vi "start_vlc_1.vi"(6 "Filename":string, 7 "wait until completion? (F)":bool, 8 "error in (no error)":errorcluster, 9 "Operation":T1(ring)=enum."Preview 320x240", 10 "VLC command":string="dshow:// --run-time=20 :dshow-vdev=\"\" :dshow-adev=\"none\" :dshow-caching=80 :dshow-fps=30.000000 -I http :sout=#transcode{vcodec=mp1v,vb=2048}:duplicate{dst=std{access=file,mux=mpeg1,dst=\"FILENAME.mpg\"}} vlc://quit", 11 "video_capture_dir":path) -> (0 "error out":errorcluster, 1 "standard output":string, 3 "standard error":string)   [LabVIEW 2018]
panel:
  out "VLC command Submitted":string
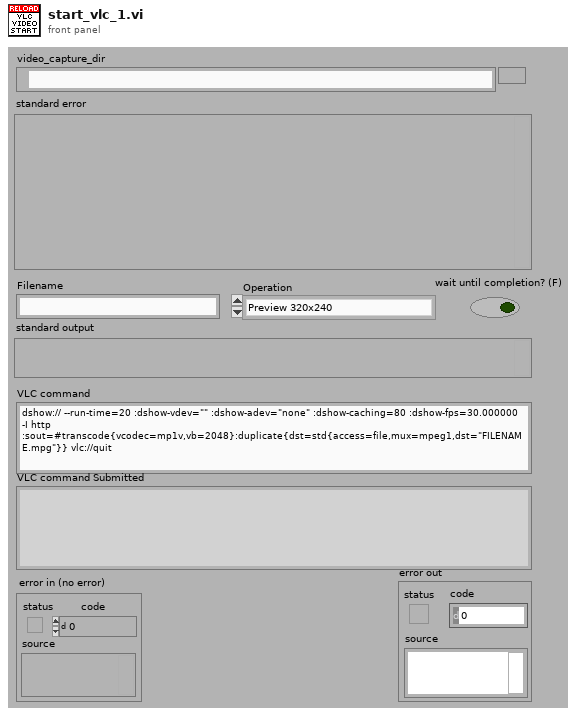
[diagram p1: front panel]
types:
  T1 = enum16{"Record to File", "Preview 320x240", "Preview 640x480"}
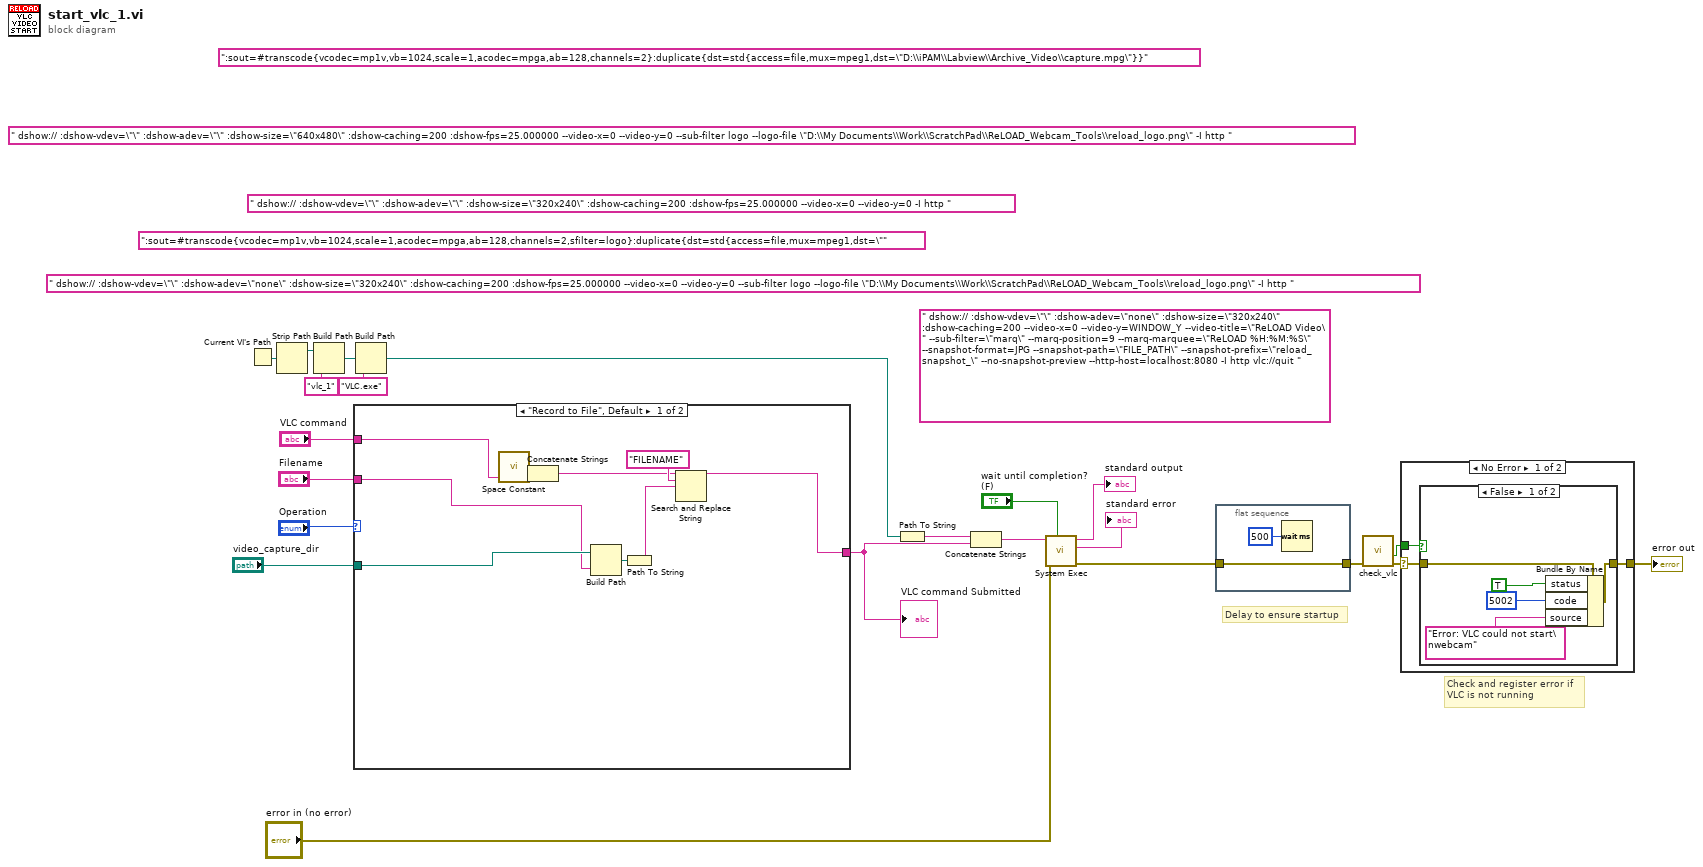
[diagram p0: block diagram]
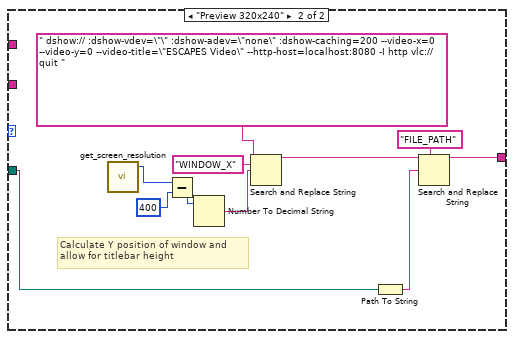
[diagram p4: hidden frame]
diagram:
  (unwired) " dshow:// :dshow-vdev=\"\" :dshow-adev=\"none\" :dshow-size=\"320x240\" :dshow-caching=200 --video-x=0 --video-y=WINDOW_Y --video-title=\"ReLOAD Video\" --sub-filter=\"marq\" --marq-position=9 --marq-marquee=\"ReLOAD %H:%M:%S\" --snapshot-format=JPG --snapshot-path=\"FILE_PATH\" --snapshot-prefix=\"reload_snapshot_\" --no-snapshot-preview --http-host=localhost:8080 -I http vlc://quit " ("Image Name")
  (unwired) ":sout=#transcode{vcodec=mp1v,vb=1024,scale=1,acodec=mpga,ab=128,channels=2}:duplicate{dst=std{access=file,mux=mpeg1,dst=\"D:\\iPAM\\Labview\\Archive_Video\\capture.mpg\"}}" ("Image Name")
  (unwired) ":sout=#transcode{vcodec=mp1v,vb=1024,scale=1,acodec=mpga,ab=128,channels=2,sfilter=logo}:duplicate{dst=std{access=file,mux=mpeg1,dst=\"" ("Image Name")
  (unwired) " dshow:// :dshow-vdev=\"\" :dshow-adev=\"none\" :dshow-size=\"320x240\" :dshow-caching=200 :dshow-fps=25.000000 --video-x=0 --video-y=0 --sub-filter logo --logo-file \"D:\\My Documents\\Work\\ScratchPad\\ReLOAD_Webcam_Tools\\reload_logo.png\" -I http " ("Image Name")
  (unwired) " dshow:// :dshow-vdev=\"\" :dshow-adev=\"\" :dshow-size=\"640x480\" :dshow-caching=200 :dshow-fps=25.000000 --video-x=0 --video-y=0 --sub-filter logo --logo-file \"D:\\My Documents\\Work\\ScratchPad\\ReLOAD_Webcam_Tools\\reload_logo.png\" -I http " ("Image Name")
  (unwired) " dshow:// :dshow-vdev=\"\" :dshow-adev=\"\" :dshow-size=\"320x240\" :dshow-caching=200 :dshow-fps=25.000000 --video-x=0 --video-y=0 -I http " ("Image Name")
  # "Check and register error if\nVLC is not running"
  # "Delay to ensure startup"
  n1 = Current VI's Path() -> (path=w16:path)
  n2 = Strip Path(path=w16) -> (stripped path=w15:path)  [unwired: 1 out]
  n3 = Build Path(base path=w15, name or relative path="vlc_1" ("search string")) -> (appended path=w13:path)
  n4 = case shown="\"Record to File\", Default" "Operation" {
    tunnel: [w23 w35] -> w10
    tunnel: "video_capture_dir" -> [w26 w36]
    tunnel: "Filename" -> [w25 _]
    tunnel: "VLC command" -> [w24 _]
    frame "Record to File", Default {
      n5 = call <vilib>:"Space Constant.vi"() -> ("String"=w27:string)
      n6 = Concatenate Strings(w27, w24) -> (w28:string)
      n7 = Build Path(base path=w26, name or relative path=w25) -> (appended path=w29:path)
      n8 = Path To String(path=w29) -> (string=w30:string)
      n9 = Search and Replace String(input string=w28, search string="FILENAME", replace string=w30) -> (result string=w23:string)  [unwired: 1 in, 7 out]
    }
    frame "Preview 320x240" {
      # "Calculate Y position of window and\nallow for titlebar height"
      n10 = call "get_screen_resolution.vi"() -> ("Width pixels"=w33:i16)  [unwired: 5 out]
      n11 = Subtract(x=w33, y=400) -> (x-y=w40:i32)
      n12 = Number To Decimal String(number=w40) -> (decimal integer string=w41:string)  [unwired: 1 out]
      n13 = Search and Replace String(input string=" dshow:// :dshow-vdev=\"\" :dshow-adev=\"none\" :dshow-caching=200 --video-x=0 --video-y=0 --video-title=\"ESCAPES Video\" --http-host=localhost:8080 -I http vlc://quit " ("Image Name"), search string="WINDOW_X", replace string=w41) -> (result string=w32:string)  [unwired: 1 in, 7 out]
      n14 = Path To String(path=w36) -> (string=w37:string)
      n15 = Search and Replace String(input string=w32, search string="FILE_PATH", replace string=w37) -> (result string=w35:string)  [unwired: 1 in, 7 out]
    }
  }
  "VLC command Submitted" <- w10
  n16 = Build Path(base path=w13, name or relative path="VLC.exe" ("search string")) -> (appended path=w12:path)
  n17 = Path To String(path=w12) -> (string=w20:string)
  n18 = Concatenate Strings(w20, w10) -> (w21:string)
  n19 = call <vilib>:"System Exec.vi"("wait until completion? (T)"="wait until completion? (F)", "error in (no error)"="error in (no error)", "command line"=w21) -> ("error out"=w3:errorcluster, "standard error"=→"standard error":string, "standard output"=→"standard output":string)  [unwired: 3 in, 3 out]
  n20 = flat-sequence {
    tunnel: w3 -> [w43]
    tunnel: [w43] -> w5
    frame #0 {
      n21 = Wait (ms)(milliseconds to wait=u32 500) -> ()  [unwired: 1 out]
    }
  }
  n22 = call "check_vlc.vi"("error in (no error)"=w5) -> ("error out"=w4:errorcluster, "Match?"=w1:bool)  [unwired: 9 out]
  n23 = case shown="No Error" w4 {
    selector: w4 -> [w46 w54]
    tunnel: [w45 w54] -> w2
    tunnel: w1 -> [w47 _]
    frame No Error {
      n24 = case shown="False" w47 {
        tunnel: w46 -> [w52 w53]
        tunnel: [w51 w53] -> w45
        frame False {
          n25 = Bundle By Name(cluster=w52, "status"=TRUE, "code"=5002, "source"="Error: VLC could not start\nwebcam") -> (w51:errorcluster)
        }
        frame True {
        }
      }
    }
    frame Error {
    }
  }
  "error out" <- w2
